vi "3DHe_Global.vi"() -> ()   [LabVIEW 2011]
panel:
  in  "optimal gain discrete":dbl[][](array[numeric])=[[6.322490035484375, 10.572770659317776, -16.036174701785043, 4.466295608355958, 3.671356663081477, -28.579439964607076, 2.2360680351129045, -1.0000002613526116], [6.322490088569187, -10.572770569940346, 16.036174259330256, 4.466295573987378, -3.6713566579553163, 28.579439419070578, 2.2360678272263246, 1.0000002101269605]] format="%.2f"
  in  "lh":dbl=0.177 format="%.3f"
  in  "Kf":dbl=0.625 format="%.2f"
  in  "la":dbl=0.66 format="%.2f"
  in  "Je":dbl=0.91 format="%.2f"
  in  "Jp":dbl=0.0364 format="%.4f"
  in  "Kp":dbl=0.686 format="%.3f"
  in  "Jt":dbl=0.91 format="%.2f"
  out "System":T1={"A"=[[0.0, 0.0, 0.0, 1.0, 0.0, 0.0, 0.0, 0.0], [0.0, 0.0, 0.0, 0.0, 1.0, 0.0, 0.0, 0.0], [0.0, 0.0, 0.0, 0.0, 0.0, 1.0, 0.0, 0.0], [0.0, 0.0, 0.0, 0.0, 0.0, 0.0, 0.0, 0.0], [0.0, 0.0, 0.0, 0.0, 0.0, 0.0, 0.0, 0.0], [0.0, -0.4975384615384616, 0.0, 0.0, 0.0, 0.0, 0.0, 0.0], [1.0, 0.0, 0.0, 0.0, 0.0, 0.0, 0.0, 0.0], [0.0, 0.0, 1.0, 0.0, 0.0, 0.0, 0.0, 0.0]], "B"=[[0.0, 0.0], [0.0, 0.0], [0.0, 0.0], [0.4532967032967033, 0.4532967032967033], [3.0391483516483517, -3.0391483516483517], [0.0, 0.0], [0.0, 0.0], [0.0, 0.0]], "C"=[[1.0, 0.0, 0.0, 0.0, 0.0, 0.0, 0.0, 0.0], [0.0, 1.0, 0.0, 0.0, 0.0, 0.0, 0.0, 0.0], [0.0, 0.0, 1.0, 0.0, 0.0, 0.0, 0.0, 0.0], [0.0, 0.0, 0.0, 1.0, 0.0, 0.0, 0.0, 0.0], [0.0, 0.0, 0.0, 0.0, 1.0, 0.0, 0.0, 0.0], [0.0, 0.0, 0.0, 0.0, 0.0, 1.0, 0.0, 0.0], [0.0, 0.0, 0.0, 0.0, 0.0, 0.0, 1.0, 0.0], [0.0, 0.0, 0.0, 0.0, 0.0, 0.0, 0.0, 1.0]], "D"=[[0.0, 0.0], [0.0, 0.0], [0.0, 0.0], [0.0, 0.0], [0.0, 0.0], [0.0, 0.0], [0.0, 0.0], [0.0, 0.0]]} {"D" format="%.2f"; "C" format="%.2f"; "B" format="%.2f"; "A" format="%.2f"}
  in  "optimal gain":dbl[][](array[numeric])=[[6.322490035484375, 10.572770659317776, -16.036174701785043, 4.466295608355958, 3.671356663081477, -28.579439964607076, 2.2360680351129045, -1.0000002613526116], [6.322490088569187, -10.572770569940346, 16.036174259330256, 4.466295573987378, -3.6713566579553163, 28.579439419070578, 2.2360678272263246, 1.0000002101269605]] format="%.2f"
  out "Kep [V/deg]":dbl=-0.22184175656234317 format="%.2f"
  out "Ked [V/ deg sec^-1]":dbl=-0.15671212600602344 format="%.2f"
  out "Kei [V/deg sec]":dbl=-0.07845852390068822 format="%.2f"
  out "Kpp [V/deg]":dbl=-0.3709744075308442 format="%.2f"
  out "Kpd [V/deg sec^-1]":dbl=-0.12881953194801393 format="%.2f"
  out "Kpi":dbl format="%.2f"
  out "Ktp [deg/deg]":dbl=1.5167428732795096 format="%.2f"
  out "Ktd [deg/deg sec^-1]":dbl=2.7031173505547126 format="%.2f"
  out "Kti [deg/deg sec]":dbl=0.09458260962893977 format="%.2f"
  # "parameters"
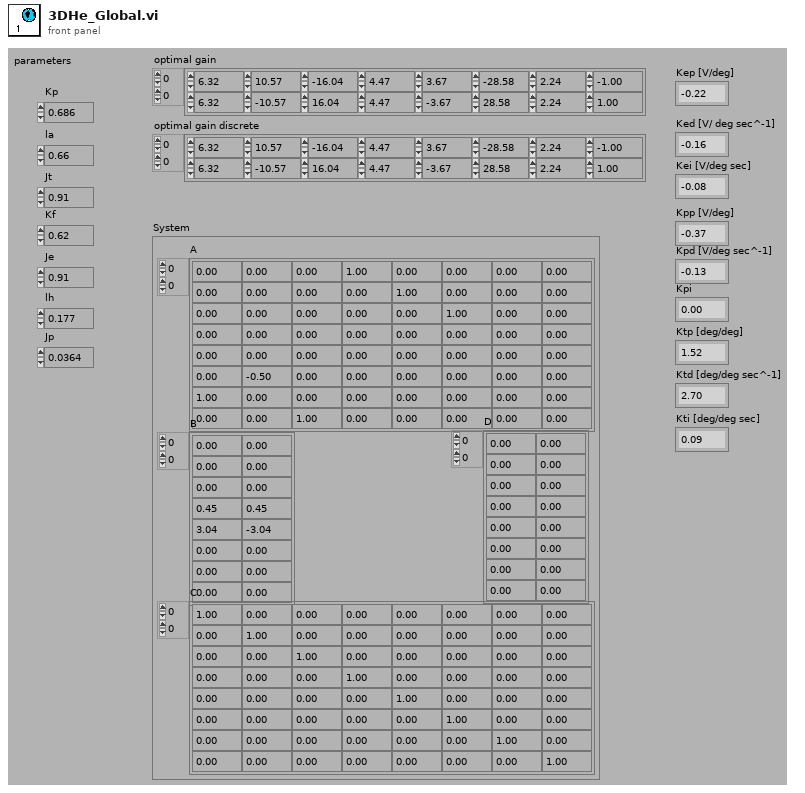
[diagram p1: front panel]
types:
  T1 = cluster{"A":dbl[][], "B":dbl[][], "C":dbl[][], "D":dbl[][]}
diagram:
